vi "CS Control.vi"() -> ()   [LabVIEW 2020]
uses:
  <instrlib>/tio-labview/TIO Library/TIO Stream Open.vi
  <instrlib>/tio-labview/TIO Library/TIO RPC Send REQuest.vi
  <instrlib>/tio-labview/TIO Library/TIO RPC Parse Reply.vi
  <instrlib>/tio-labview/TIO Library/TIO RPC Parse Reply Error.vi
  <instrlib>/tio-labview/TIO Library/TIO Data Stream Parse timebase Info.vi
  <instrlib>/tio-labview/TIO Library/TIO Data Stream Parse pstream Info.vi
  <instrlib>/tio-labview/TIO Library/TIO Data Stream Parse dstream Info.vi
  <vilib>/Utility/High Resolution Relative Seconds.vi
  <instrlib>/tio-labview/TIO Library/TIO RPC Notification.vi
  <vilib>/Utility/error.llb/Clear Errors.vi
  <instrlib>/tio-labview/TIO Library/TIO Serial Port Name Search.vi
  <instrlib>/tio-labview/TIO Library/TIO Stream Write.vi
  <instrlib>/tio-labview/TIO Library/TIO RPC Form Request.vi
  <instrlib>/tio-labview/TIO Library/TIO SLIP Serial Write.vi
  <instrlib>/tio-labview/TIO Library/TIO Form Packet.vi
  <instrlib>/tio-labview/TIO Library/TIO SLIP Encode.vi
  <instrlib>/tio-labview/TIO Library/TIO Serial Checksum CRC32.vi
  <vilib>/Utility/tcp.llb/UDP Multicast Open.vi
  <vilib>/Utility/tcp.llb/UDP Multicast Read-Write Open.vi
  <instrlib>/tio-labview/TIO Library/TIO Serial Port Discovery.vi
  <vilib>/Instr/_visa.llb/VISA Configure Serial Port (Instr).vi
  <instrlib>/tio-labview/TIO Library/TIO RPC Blocking.vi
  <instrlib>/tio-labview/TIO Library/TIO Stream Read Non-blocking.vi
  <instrlib>/tio-labview/TIO Library/TIO RPC Send Heartbeat.vi
panel:
  in  "Quit 2":bool
  in  "X":dbl[unit](slide)
  in  "Y":dbl[unit](slide)
  in  "Z":dbl[unit](slide)
  in  "Quit":bool
  out "ID":string
  in  "URL":refnum<visa-resource-name>="tcp://localhost"
  # "CSB Control"
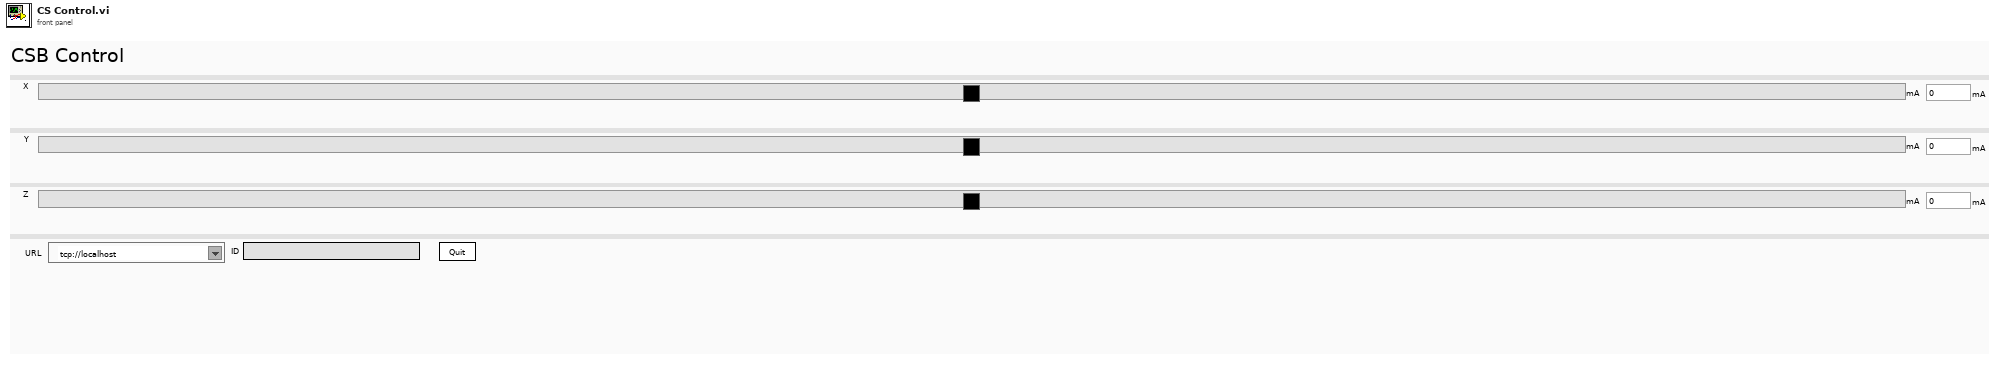
[diagram p1: front panel]
types:
  T1 = cluster{"TS Connection":cluster{"Type":enum16{"Serial", "TCP", "UDP", "mUDP"}, "URL":refnum<visa-resource-name>, "TO":u32, "Addr":u32, "Port":i32, "TCP":refnum<k5>, "UDP":refnum<k16>, "Route":string}, "REQ":refnum<queue>, "REP":refnum<queue>}
  T2 = cluster{"Awaiting REP":bool, "REQ ID":u32, "streams in":cluster{"id":u16, "timebase id":u16, "period":u32, "offset":u32, "sample number":u64, "total components":u16, "flags":u16, "components":cluster{"source id":u16, "flags":u16, "period":u32, "offset":u32}[]}[], "sources":cluster{"id":u16, "timebase_id":u16, "period":u32, "offset":u32, "fmt":i32, "flags":u16, "channels":u16, "type":u8, "name":string, "column names":string[], "title":string, "units":string}[], "timebases":cluster{"id":u16, "source":u8, "epoch":u8, "start time":u64, "period numerator (µs)":u32, "period denominator (µs)":u32, "flags":u32, "stability":sgl, "source id":string}[]}
  T3 = cluster{"TC Connection":cluster{"Type":enum16{"Serial", "TCP", "UDP", "mUDP"}, "URL":refnum<visa-resource-name>, "TO":u32, "Addr":u32, "Port":i32, "TCP":refnum<k5>, "UDP":refnum<k16>, "Route":string}, "REQ":refnum<queue>, "REP":refnum<queue>}
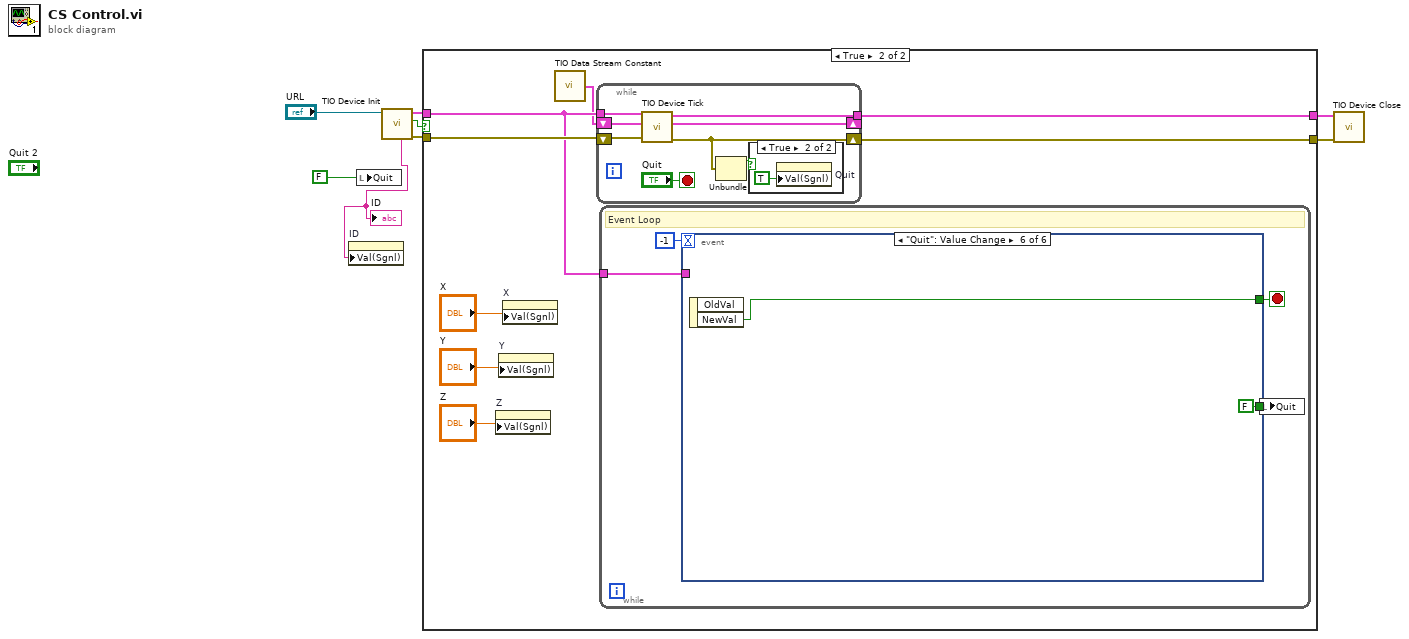
[diagram p0: block diagram]
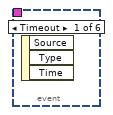
[diagram p4: hidden frame]
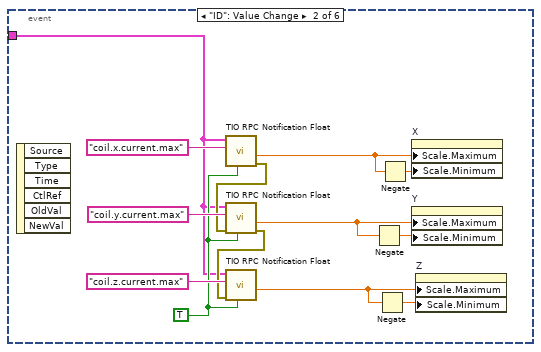
[diagram p5: hidden frame]
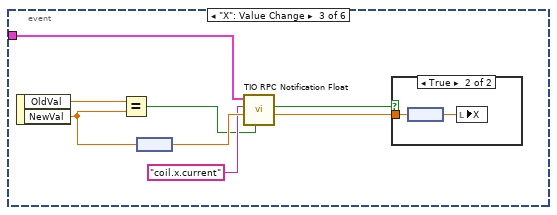
[diagram p6: hidden frame]
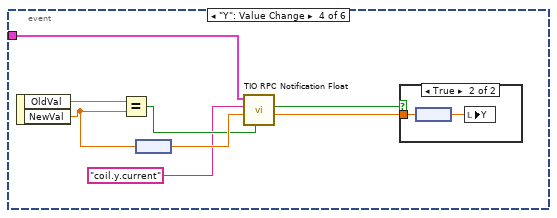
[diagram p8: hidden frame]
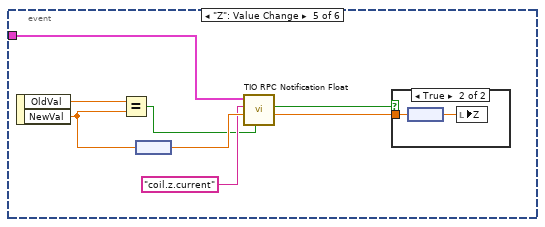
[diagram p10: hidden frame]
diagram:
  n1 = local write "Quit"(FALSE ("Quit")) -> ()
  n2 = call <instrlib>:"TIO Device Init.vi"("URL"="URL") -> ("error out"=w5:errorcluster, 2:"ID Verified"=w6:bool, "TIO"=w7:T1, 4:"ID Verified"=w1:string)  [unwired: 6 in, 1 out]
  "ID" <- w1
  n3 = property on="ID" class="Str"("Val(Sgnl)"=w1) -> ()  [unwired: 2 in, 2 out]
  n4 = case shown="True" w6 {
    tunnel: w7 -> [w10 w14]
    tunnel: w5 -> [w9 w15]
    tunnel: [w9 w13] -> w3
    tunnel: [w10 w12] -> w2
    frame False {
    }
    frame True {
      n5 = property on="Z" class="Slide (strict)"("Val(Sgnl)"="Z") -> ()  [unwired: 2 in, 2 out]
      n6 = property on="Y" class="Slide (strict)"("Val(Sgnl)"="Y") -> ()  [unwired: 2 in, 2 out]
      n7 = property on="X" class="Slide (strict)"("Val(Sgnl)"="X") -> ()  [unwired: 2 in, 2 out]
      n8 = call <instrlib>:"TIO Data Stream Constant.vi"() -> ("TIO State"=w11:T2)
      n9 = while {
        tunnel: w14 -> [w25]
        shift-right: [w23] -> _
        shift-left: w11 -> [w22]
        tunnel: [w21] -> w12
        shift-right: [w20] -> w13
        shift-left: w15 -> [w26]
        stop <- "Quit" stop-if-true
        n10 = call <instrlib>:"TIO Device Tick.vi"("Error in"=w26, "TIO State"=w22, "TIO"=w25) -> ("Error out"=w20:errorcluster, "TIO State"=w23:T2, "TIO"=w21:T3)  [unwired: 5 in, 1 out]
        n11 = Unbundle(w20) -> ("status"=w19:bool)  [unwired: 2 out]
        n12 = case shown="True" w19 {
          frame False {
          }
          frame True {
            n13 = property on="Quit" class="Bool (strict)"("Val(Sgnl)"=TRUE ("Value (Signaling)")) -> ()  [unwired: 2 in, 2 out]
          }
        }
      }
      n14 = while {
        tunnel: w14 -> [w30]
        stop <- w29 stop-if-true
        # "Event Loop"
        n15 = event shown="[5] \"Quit\": Value Change" {
          selector: _ -> [_ _ _ _ _ _]
          dyn-events: _ -> [_ _ _ _ _ _]
          timeout: -1 -> [_ _ _ _ _ _]
          tunnel: w30 -> [_ w32 w47 w56 w65 _]
          tunnel: [_ _ _ _ _ w76] -> w29
          tunnel: [_ _ _ _ _ FALSE ("Quit")] -> w28
          event Timeout {
            n16 = event-data() -> ()  [unwired: 1 in, 3 out]
          }
          event "ID": Value Change {
            w33 = TRUE ("Read")
            n17 = event-data() -> ()  [unwired: 1 in, 6 out]
            n18 = call <instrlib>:"TIO RPC Notification Float.vi"("Read"=w33, "Topic"="coil.x.current.max", "TIO"=w32) -> ("error out"=w37:errorcluster, "Get value (default if error)"=w39:sgl)  [unwired: 5 in, 1 out]
            n19 = call <instrlib>:"TIO RPC Notification Float.vi"("Read"=w33, "error in (no error)"=w37, "Topic"="coil.y.current.max", "TIO"=w32) -> ("error out"=w34:errorcluster, "Get value (default if error)"=w36:sgl)  [unwired: 4 in, 1 out]
            n20 = call <instrlib>:"TIO RPC Notification Float.vi"("Read"=w33, "error in (no error)"=w34, "Topic"="coil.z.current.max", "TIO"=w32) -> ("Get value (default if error)"=w35:sgl)  [unwired: 4 in, 2 out]
            n21 = Negate(x=w36) -> (-x=w44:sgl)
            n22 = Negate(x=w35) -> (-x=w43:sgl)
            n23 = Negate(x=w39) -> (-x=w38:sgl)
            n24 = property on="X" class="Slide (strict)"("Scale.Maximum"=w39, "Scale.Minimum"=w38) -> ()  [unwired: 2 in, 2 out]
            n25 = property on="Y" class="Slide (strict)"("Scale.Maximum"=w36, "Scale.Minimum"=w44) -> ()  [unwired: 2 in, 2 out]
            n26 = property on="Z" class="Slide (strict)"("Scale.Maximum"=w35, "Scale.Minimum"=w43) -> ()  [unwired: 2 in, 2 out]
          }
          event "X": Value Change {
            n27 = event-data() -> ("OldVal"=w49:dbl[unit], "NewVal"=w48:dbl[unit])  [unwired: 1 in]
            n28 = Equal?(x=w49, y=w48) -> (x = y?=w45:bool)
            n29 = node(w48) -> (w52:dbl)
            n30 = call <instrlib>:"TIO RPC Notification Float.vi"("Read"=w45, "Set value"=w52, "Topic"="coil.x.current", "TIO"=w47) -> ("Get value (default if error)"=w51:sgl, "Response"=w50:bool)  [unwired: 4 in, 1 out]
            n31 = case shown="True" w50 {
              tunnel: w51 -> [_ w54]
              frame False {
              }
              frame True {
                n32 = node(w54) -> (w53:sgl[unit])
                n33 = local write "X"(w53) -> ()
              }
            }
          }
          event "Y": Value Change {
            n34 = event-data() -> ("OldVal"=w59:dbl[unit], "NewVal"=w58:dbl[unit])  [unwired: 1 in]
            n35 = Equal?(x=w59, y=w58) -> (x = y?=w57:bool)
            n36 = node(w58) -> (w62:dbl)
            n37 = call <instrlib>:"TIO RPC Notification Float.vi"("Read"=w57, "Set value"=w62, "Topic"="coil.y.current", "TIO"=w56) -> ("Get value (default if error)"=w61:sgl, "Response"=w60:bool)  [unwired: 4 in, 1 out]
            n38 = case shown="True" w60 {
              tunnel: w61 -> [_ w64]
              frame False {
              }
              frame True {
                n39 = node(w64) -> (w63:sgl[unit])
                n40 = local write "Y"(w63) -> ()
              }
            }
          }
          event "Z": Value Change {
            n41 = event-data() -> ("OldVal"=w69:dbl[unit], "NewVal"=w68:dbl[unit])  [unwired: 1 in]
            n42 = Equal?(x=w69, y=w68) -> (x = y?=w66:bool)
            n43 = node(w68) -> (w72:dbl)
            n44 = call <instrlib>:"TIO RPC Notification Float.vi"("Read"=w66, "Set value"=w72, "Topic"="coil.z.current", "TIO"=w65) -> ("Get value (default if error)"=w71:sgl, "Response"=w70:bool)  [unwired: 4 in, 1 out]
            n45 = case shown="True" w70 {
              tunnel: w71 -> [_ w74]
              frame False {
              }
              frame True {
                n46 = node(w74) -> (w73:sgl[unit])
                n47 = local write "Z"(w73) -> ()
              }
            }
          }
          event "Quit": Value Change {
            n48 = event-data() -> ("NewVal"=w76:bool)  [unwired: 1 in, 1 out]
          }
        }
        n49 = local write "Quit"(w28) -> ()
      }
    }
  }
  n50 = call <instrlib>:"TIO Device Close.vi"("Error in"=w3, "TIO"=w2) -> ()  [unwired: 10 in]
